vi "Get Object Data.vi"(8 "error in (no error)":errorcluster, 10 "Object DAO":refnum<class "Object DAO.lvclass">) -> (0 "error out":errorcluster, 1 "ids":string[](array[string]), 2 "Objects":refnum<class "iObject.lvclass">[](array[class]))   [LabVIEW 2020, in "Object DAO Adapter.lvclass"]
uses:
  Object DAO Adapter.lvclass
  Object DAO/Object DAO.lvclass
  iObject/iObject.lvclass
  Object DAO/Object DAO.lvclass/Object DAO.ctl
  Object/Object.lvclass
  C:/Users/fflores/Desktop/DataBase - Copy - Copy/iOrder/iObject.lvclass
  Object/Object.lvclass/Object.ctl
  Object/Member Accessors/Set String.vi
  Object/Member Accessors/Set Boolean.vi
  Object/Member Accessors/Set Numeric.vi
  Object DAO/Member Accessors/Get Retrieved Items.vi
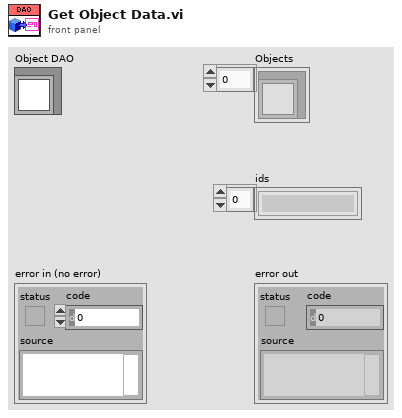
[diagram p1: front panel]
types:
  T1 = typedef "Object DAO.lvclass/Object Information.ctl" = cluster{"String":string, "Boolean":bool, "Numeric":dbl, "id":string}
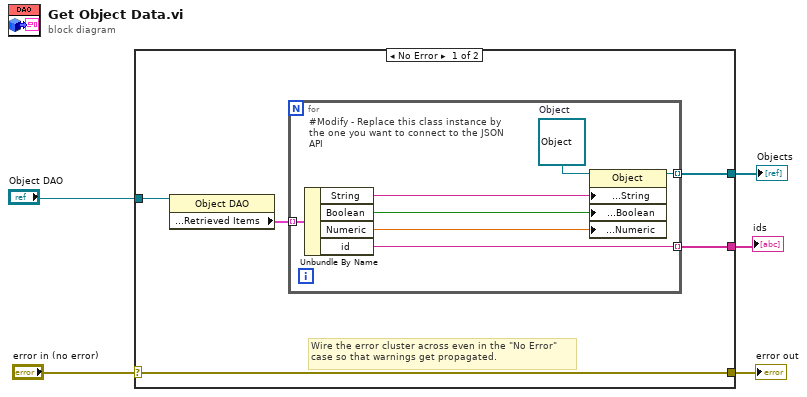
[diagram p0: block diagram]
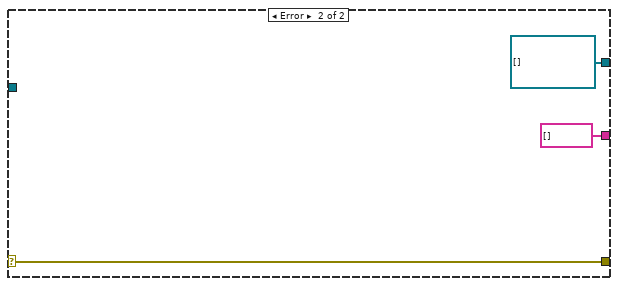
[diagram p2: hidden frame]
diagram:
  n1 = case shown="No Error" "error in (no error)" {
    selector: "error in (no error)" -> [w10 w20]
    tunnel: [w10 w20] -> w4
    tunnel: "Object DAO" -> [w9 _]
    tunnel: [w7 refnum<class "Object.lvclass">[] [] ("Array")] -> w2
    tunnel: [w6 string[] []] -> w1
    frame No Error {
      # "Wire the error cluster across even in the \"No Error\"\ncase so that warnings get propagated."
      n2 = property class="Object DAO"(reference=w9) -> ("Member Accessors:Retrieved Items"=w8:T1[])  [unwired: 1 in, 2 out]
      n3 = for {
        tunnel: w8 -> [w17] mode=indexing
        tunnel: [w12] -> w7 mode=indexing
        tunnel: [w11] -> w6 mode=indexing
        w16 = refnum<class "Object.lvclass"> refnum  # Object
        # "#Modify - Replace this class instance by the one you want to connect to the JSON API"
        n4 = Unbundle By Name(w17) -> ("String"=w15:string, "Boolean"=w14:bool, "Numeric"=w13:dbl, "id"=w11:string)
        n5 = property class="Object"(reference=w16, "Member Accessors:String"=w15, "Member Accessors:Boolean"=w14, "Member Accessors:Numeric"=w13) -> (reference out=w12:refnum<class "Object.lvclass">)  [unwired: 1 in, 1 out]
      }
    }
    frame Error {
    }
  }
  "error out" <- w4
  "Objects" <- w2
  "ids" <- w1
